vi "Rearrane images2.vi"(0 "Selet tab":enum16{"Diagnostics", "Main"}(ring), 1 "Image indicator layouts 2":T1(array[cluster])=[{"NumberOfImageIndicators"=0.0, "ImageSpecificData"=[{"Width"=0.0, "Left"=0.0, "Top"=0.0, "Image Percentage"={"Height"=0.0, "Width correction"=0.0, "Height correction"=0.0, "Left correction"=0.0, "Top correction"=0.0}, "String Percentage"={"Height"=0.0, "Width correction"=0.0, "Height correction"=0.0, "Left correction"=0.0, "Top correction"=0.0}}, {"Width"=0.0, "Left"=0.0, "Top"=0.0, "Image Percentage"={"Height"=0.0, "Width correction"=0.0, "Height correction"=0.0, "Left correction"=0.0, "Top correction"=0.0}, "String Percentage"={"Height"=0.0, "Width correction"=0.0, "Height correction"=0.0, "Left correction"=0.0, "Top correction"=0.0}}, {"Width"=0.5, "Left"=0.0, "Top"=0.0, "Image Percentage"={"Height"=0.45, "Width correction"=-10.0, "Height correction"=0.0, "Left correction"=0.0, "Top correction"=0.0}, "String Percentage"={"Height"=0.05, "Width correction"=-5.0, "Height correction"=0.0, "Left correction"=0.0, "Top correction"=0.0}}, {"Width"=0.5, "Left"=0.0, "Top"=0.5, "Image Percentage"={"Height"=0.0, "Width correction"=-10.0, "Height correction"=0.0, "Left correction"=0.0, "Top correction"=0.0}, "String Percentage"={"Height"=0.0, "Width correction"=-5.0, "Height correction"=0.0, "Left correction"=0.0, "Top correction"=0.0}}, {"Width"=0.5, "Left"=0.5, "Top"=0.0, "Image Percentage"={"Height"=0.95, "Width correction"=-10.0, "Height correction"=0.0, "Left correction"=0.0, "Top correction"=0.0}, "String Percentage"={"Height"=0.05, "Width correction"=-5.0, "Height correction"=0.0, "Left correction"=0.0, "Top correction"=0.0}}]}, {"NumberOfImageIndicators"=0.0, "ImageSpecificData"=[]}, {"NumberOfImageIndicators"=0.0, "ImageSpecificData"=[{"Width"=0.5, "Left"=0.0, "Top"=0.0, "Image Percentage"={"Height"=0.45, "Width correction"=-7.0, "Height correction"=0.0, "Left correction"=0.0, "Top correction"=0.0}, "String Percentage"={"Height"=0.05, "Width correction"=-5.0, "Height correction"=0.0, "Left correction"=0.0, "Top correction"=0.0}}, {"Width"=0.5, "Left"=0.0, "Top"=0.5, "Image Percentage"={"Height"=0.45, "Width correction"=-7.0, "Height correction"=0.0, "Left correction"=0.0, "Top correction"=0.0}, "String Percentage"={"Height"=0.05, "Width correction"=-5.0, "Height correction"=0.0, "Left correction"=0.0, "Top correction"=0.0}}, {"Width"=0.5, "Left"=0.5, "Top"=0.0, "Image Percentage"={"Height"=0.95, "Width correction"=-7.0, "Height correction"=0.0, "Left correction"=0.0, "Top correction"=0.0}, "String Percentage"={"Height"=0.05, "Width correction"=-5.0, "Height correction"=0.0, "Left correction"=0.0, "Top correction"=0.0}}, {"Width"=0.5, "Left"=0.0, "Top"=0.5, "Image Percentage"={"Height"=0.45, "Width correction"=-7.0, "Height correction"=0.0, "Left correction"=0.0, "Top correction"=0.0}, "String Percentage"={"Height"=0.05, "Width correction"=-5.0, "Height correction"=0.0, "Left correction"=0.0, "Top correction"=0.0}}, {"Width"=0.5, "Left"=0.5, "Top"=0.0, "Image Percentage"={"Height"=0.0, "Width correction"=-7.0, "Height correction"=0.0, "Left correction"=0.0, "Top correction"=0.0}, "String Percentage"={"Height"=0.0, "Width correction"=-5.0, "Height correction"=0.0, "Left correction"=0.0, "Top correction"=0.0}}]}], 2 "Update\nTables":bool=TRUE, 5 "Camera names":string[](array[string]), 7 "Type of label":u16(ring) items=["Combo", "String"], 9 "References":T2, 11 "error in (no error)":errorcluster, 12 "Table column headers":string[](array[string])) -> (15 "error out":errorcluster)   [LabVIEW 2015]
uses:
  <vilib>/Utility/miscctls.llb/LVRowAndColumnTypeDef.ctl
  E:/Test codes/User Interface Testbench/May backups/Test bench (05-05-2018)/User Interface/User Interface Actor/ZenGage v3.0 UI.lvclass
panel:
  in  "#Racks":u8
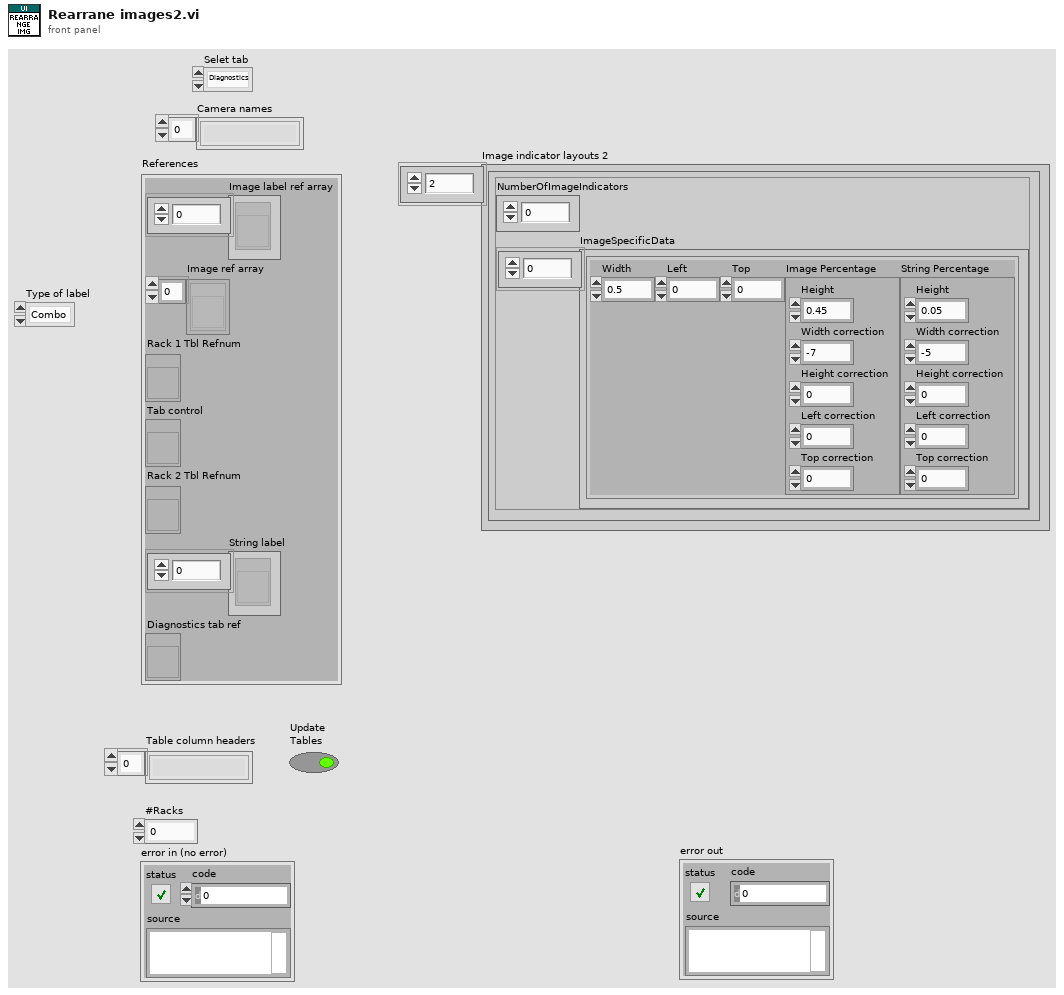
[diagram p1: front panel]
types:
  T1 = cluster{"NumberOfImageIndicators":dbl, "ImageSpecificData":cluster{"Width":dbl, "Left":dbl, "Top":dbl, "Image Percentage":cluster{"Height":dbl, "Width correction":dbl, "Height correction":dbl, "Left correction":dbl, "Top correction":dbl}, "String Percentage":cluster{"Height":dbl, "Width correction":dbl, "Height correction":dbl, "Left correction":dbl, "Top correction":dbl}}[]}[]
  T2 = cluster{"Image label ref array":refnum<vi>[], "Image ref array":refnum<vi>[], "Rack 1 Tbl Refnum":refnum<vi>, "Tab control":refnum<vi>, "Rack 2 Tbl Refnum":refnum<vi>, "String label":refnum<vi>[], "Diagnostics tab ref":refnum<vi>}
  T3 = cluster{"NumberOfImageIndicators":dbl, "ImageSpecificData":cluster{"Width":dbl, "Left":dbl, "Top":dbl, "Image Percentage":cluster{"Height":dbl, "Width correction":dbl, "Height correction":dbl, "Left correction":dbl, "Top correction":dbl}, "String Percentage":cluster{"Height":dbl, "Width correction":dbl, "Height correction":dbl, "Left correction":dbl, "Top correction":dbl}}[]}
  T4 = cluster{"Width":dbl, "Left":dbl, "Top":dbl, "Image Percentage":cluster{"Height":dbl, "Width correction":dbl, "Height correction":dbl, "Left correction":dbl, "Top correction":dbl}, "String Percentage":cluster{"Height":dbl, "Width correction":dbl, "Height correction":dbl, "Left correction":dbl, "Top correction":dbl}}[]
  T5 = typedef "LVRowAndColumnTypeDef.ctl" = cluster{"Row":i32, "Column":i32}
  T6 = cluster{"Tab width":u32, "Tab height":u32, "Left":i32, "Top":i32}
  T7 = cluster{"Width":dbl, "Left":dbl, "Top":dbl, "Image Percentage":cluster{"Height":dbl, "Width correction":dbl, "Height correction":dbl, "Left correction":dbl, "Top correction":dbl}, "String Percentage":cluster{"Height":dbl, "Width correction":dbl, "Height correction":dbl, "Left correction":dbl, "Top correction":dbl}}
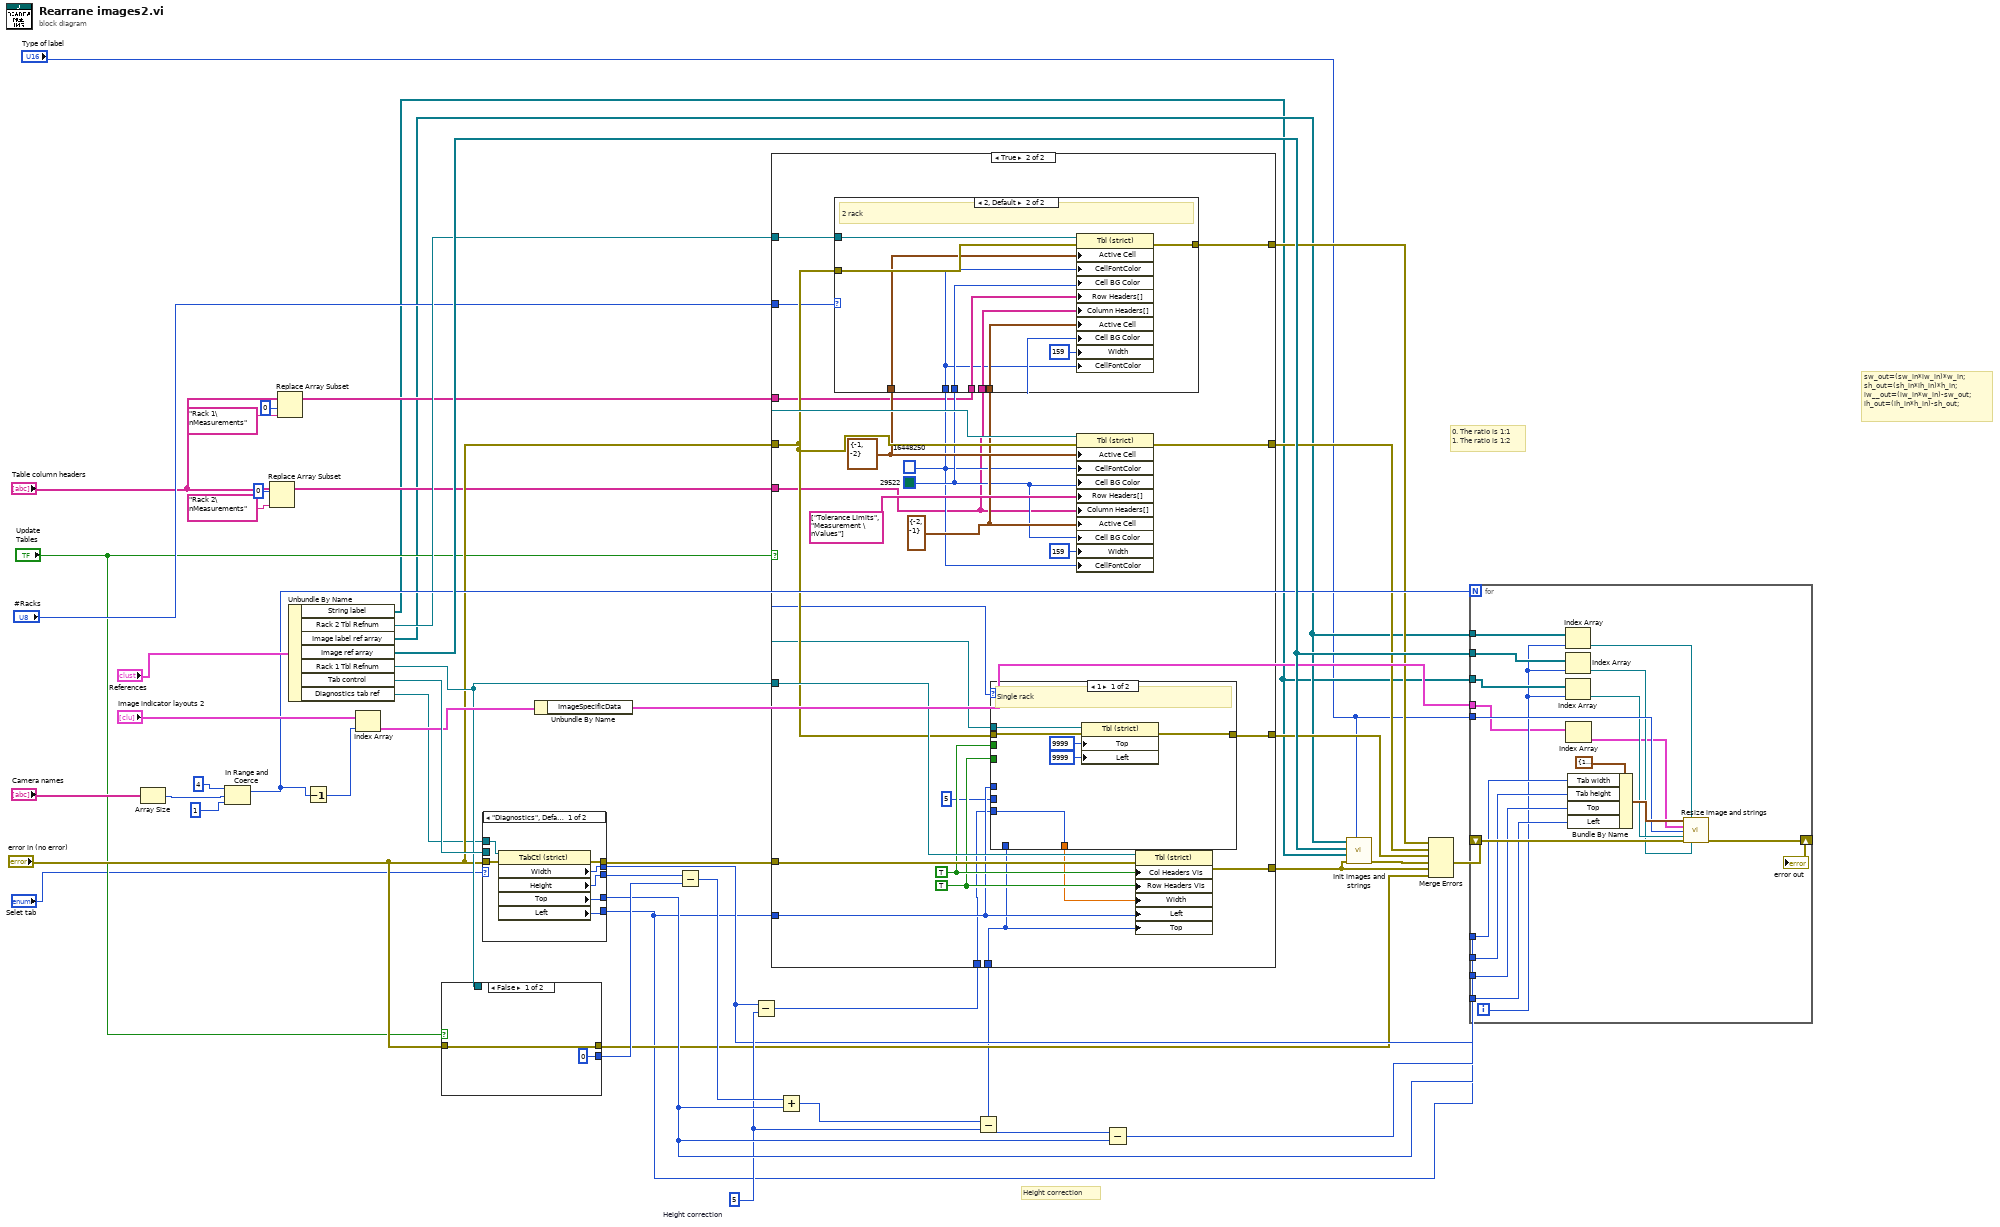
[diagram p0: block diagram]
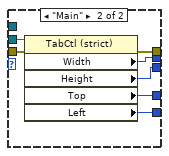
[diagram p2: hidden frame]
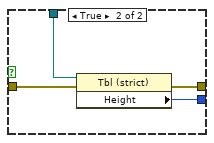
[diagram p3: hidden frame]
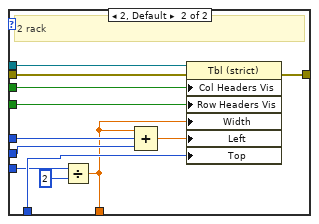
[diagram p5: hidden frame]
diagram:
  w39 = u32 5  # Height correction
  # "Height correction"
  # "sw_out=(sw_in*iw_in)*w_in;\nsh_out=(sh_in*ih_in)*h_in;\niw__out=(iw_in*w_in)-sw_out;\nih_out=(ih_in*h_in)-sh_out;"
  # "0. The ratio is 1:1\n1. The ratio is 1:2"
  n1 = Array Size(array="Camera names") -> (size(s)=w25:i32)
  n2 = In Range and Coerce(upper limit=4 ("size(s)"), x=w25, lower limit=1 ("size(s)")) -> (coerced(x)=w24:i32)  [unwired: 1 out]
  n3 = Replace Array Subset(array="Table column headers", new element="Rack 2\nMeasurements" ("new element/subarray"), index=0) -> (w13:string[])
  n4 = Replace Array Subset(array="Table column headers", new element="Rack 1\nMeasurements" ("new element/subarray"), index=0) -> (w12:string[])
  n5 = Unbundle By Name("References") -> ("String label"=w4:refnum<vi>[], "Rack 2 Tbl Refnum"=w17:refnum<vi>, "Image label ref array"=w6:refnum<vi>[], "Image ref array"=w42:refnum<vi>[], "Rack 1 Tbl Refnum"=w34:refnum<vi>, "Tab control"=w41:refnum<vi>, "Diagnostics tab ref"=w1:refnum<vi>)
  n6 = Decrement(x=w24) -> (x-1=w29:i32)
  n7 = Index Array(array="Image indicator layouts 2", index=w29) -> (element=w36:T3)
  n8 = case shown="False" "Update\nTables" {
    tunnel: [u32 0 ("Height") w55] -> w47
    tunnel: w34 -> [_ w54]
    tunnel: [w51 w53] -> w30
    tunnel: "error in (no error)" -> [w51 w52]
    frame False {
    }
    frame True {
      n9 = property on="Property Node" class="Tbl (strict)"(reference=w54, error in=w52) -> (error out=w53:errorcluster, "Height"=w55:u32)  [unwired: 1 out]
    }
  }
  n10 = case shown="\"Diagnostics\", Default" "Selet tab" {
    tunnel: [w58 w69] -> w44
    tunnel: w41 -> [_ w68]
    tunnel: [w59 w67] -> w40
    tunnel: [w60 w66] -> w38
    tunnel: [w61 w65] -> w33
    tunnel: "error in (no error)" -> [w62 w64]
    tunnel: [w57 w63] -> w19
    tunnel: w1 -> [w56 _]
    frame "Diagnostics", Default {
      n11 = property class="TabCtl (strict)"(reference=w56, error in=w62) -> (error out=w61:errorcluster, "Width"=w60:u32, "Height"=w59:u32, "Top"=w58:i32, "Left"=w57:i32)  [unwired: 1 out]
    }
    frame "Main" {
      n12 = property class="TabCtl (strict)"(reference=w68, error in=w64) -> (error out=w65:errorcluster, "Width"=w66:u32, "Height"=w67:u32, "Top"=w69:i32, "Left"=w63:i32)  [unwired: 1 out]
    }
  }
  n13 = Unbundle By Name(w36) -> ("ImageSpecificData"=w35:T4)
  n14 = Subtract(x=w40, y=w47) -> (x-y=w49:u32)
  n15 = Subtract(x=w38, y=w39) -> (x-y=w16:u32)
  n16 = Add(x=w49, y=w44) -> (x+y=w48:u32)
  n17 = Subtract(x=w48, y=w39) -> (x-y=w18:u32)
  n18 = case shown="True" "Update\nTables" {
    tunnel: w34 -> [_ w94]
    tunnel: w33 -> [w70 w93]
    tunnel: [w71 w92] -> w23
    tunnel: [w70 w91] -> w22
    tunnel: "error in (no error)" -> [w71 w90]
    tunnel: [w71 w84] -> w20
    tunnel: w19 -> [_ w81]
    tunnel: w18 -> [_ w79]
    tunnel: [w70 w78] -> w5
    tunnel: w17 -> [_ w77]
    tunnel: w16 -> [_ w76]
    tunnel: "#Racks" -> [_ w74]
    tunnel: w13 -> [_ w73]
    tunnel: w12 -> [_ w72]
    frame False {
    }
    frame True {
      w87 = T5 {"Row"=-2, "Column"=-1} ("Active Cell:Active Cell")
      w89 = T5 {"Row"=-1, "Column"=-2} ("Active Cell:Active Cell")
      w86 = u32 29522
      w85 = u32 16448250
      w82 = TRUE ("Visible Items:Row Headers Visible")
      w83 = TRUE ("Visible Items:Column Headers Visible")
      n19 = case shown="2, Default" w74 {
        tunnel: w90 -> [w114 w123]
        tunnel: w89 -> [_ w122]
        tunnel: w72 -> [_ w121]
        tunnel: w73 -> [_ w120]
        tunnel: w87 -> [_ w119]
        tunnel: w86 -> [_ w118]
        tunnel: w85 -> [_ w117]
        tunnel: [w114 w116] -> w84
        tunnel: w77 -> [_ w115]
        frame 1 {
          # "Single rack"
        }
        frame 2, Default {
          # "2 rack"
          n20 = property class="Tbl (strict)"(reference=w115, error in=w123, "Active Cell"=w122, "CellFontColor"=w117, "Cell BG Color"=w118, "Row Headers[]"=w121, "Column Headers[]"=w120, "Active Cell"=w119, "Cell BG Color"=w118, "Width"=u32 159 ("Active Cell:Cell Size:Width"), "CellFontColor"=w117) -> (error out=w116:errorcluster)  [unwired: 1 out]
        }
      }
      n21 = case shown="1" w74 {
        tunnel: [w99 w113] -> w91
        tunnel: w90 -> [w100 w112]
        tunnel: w83 -> [_ w111]
        tunnel: w82 -> [_ w110]
        tunnel: w81 -> [_ w109]
        tunnel: 5 ("value") -> [_ w108]
        tunnel: w79 -> [_ w106]
        tunnel: w77 -> [w96 w105]
        tunnel: w76 -> [w101 w104]
        tunnel: [w101 w102] -> w75
        frame 1 {
          # "Single rack"
          n22 = property on="Property Node" class="Tbl (strict)"(reference=w96, error in=w100, "Top"=9999 ("Position:Top"), "Left"=9999 ("Position:Left")) -> (error out=w99:errorcluster)  [unwired: 1 out]
        }
        frame 2, Default {
          # "2 rack"
          n23 = Divide(x=w104, y=u32 2) -> (x/y=w102:dbl)
          n24 = Compound Arithmetic op=ADD(w102, w109, w108) -> (w107:dbl)
          n25 = property on="Property Node" class="Tbl (strict)"(reference=w105, error in=w112, "Col Headers Vis"=w111, "Row Headers Vis"=w110, "Width"=w102, "Left"=w107, "Top"=w106) -> (error out=w113:errorcluster)  [unwired: 1 out]
        }
      }
      n26 = property class="Tbl (strict)"(reference=w94, error in=w90, "Active Cell"=w89, "CellFontColor"=w85, "Cell BG Color"=w86, "Row Headers[]"=string[] ["Tolerance Limits", "Measurement \nValues"] ("Row Header"), "Column Headers[]"=w73, "Active Cell"=w87, "Cell BG Color"=w86, "Width"=u32 159 ("Active Cell:Cell Size:Width"), "CellFontColor"=w85) -> (error out=w92:errorcluster)  [unwired: 1 out]
      n27 = property on="Property Node" class="Tbl (strict)"(reference=w94, error in=w93, "Col Headers Vis"=w83, "Row Headers Vis"=w82, "Width"=w75, "Left"=w81, "Top"=w79) -> (error out=w78:errorcluster)  [unwired: 1 out]
    }
  }
  n28 = Subtract(x=w18, y=w44) -> (x-y=w46:u32)
  n29 = call "Init images and strings.vi"("Type of label"="Type of label", "error in (no error)"=w5, "String label"=w4, "Image ref array"=w42, "Image label ref array"=w6) -> ("error in (no error) 2"=w32:errorcluster)  [unwired: 6 in]
  n30 = Merge Errors(w20, w23, w22, w32, w5, w30) -> (w31:errorcluster)
  n31 = for {
    N: w24 -> [_]
    tunnel: w46 -> [w139]
    tunnel: w38 -> [w140]
    tunnel: w6 -> [w133]
    tunnel: w42 -> [w132]
    tunnel: w35 -> [w126]
    shift-right: [w141] -> w45
    shift-left: w31 -> [w142]
    tunnel: w19 -> [w135]
    tunnel: w44 -> [w136]
    tunnel: "Type of label" -> [w134]
    tunnel: w4 -> [w131]
    i -> [w130]
    n32 = Index Array(array=w133, index=w130) -> (element=w129:refnum<vi>)
    n33 = Index Array(array=w132, index=w130) -> (element=w127:refnum<vi>)
    n34 = Index Array(array=w131, index=w130) -> (element=w128:refnum<vi>)
    n35 = Index Array(array=w126) -> (element=w125:T7)  [unwired: 1 in]
    n36 = Bundle By Name(cluster=T6 {"Tab width"=1176, "Tab height"=619, "Left"=0, "Top"=0} ("Tab details"), "Tab width"=w140, "Tab height"=w139, "Top"=w136, "Left"=w135) -> (w137:T6)
    n37 = call "Resize image and strings.vi"("Tab details"=w137, "Image label 2"=w129, "Image position and resize"=w125, "Type of label"=w134, "String label"=w128, "error in (no error)"=w142, "Img Refnum"=w127) -> ("error out"=w141:errorcluster)  [unwired: 8 in]
  }
  "error out" <- w45
